vi "Get Cache Path.vi"(8 "error in (no error)":errorcluster, 11 "IPath Getter in":refnum<class "IPath Getter.lvclass">) -> (0 "error out":errorcluster, 2 "Path":path)   [LabVIEW 2020, in "IPath Getter.lvclass"]
doc: "Definition of input/output parameters for <b>Get Cache Path</b> implementation."
uses:
  IPath Getter.lvclass
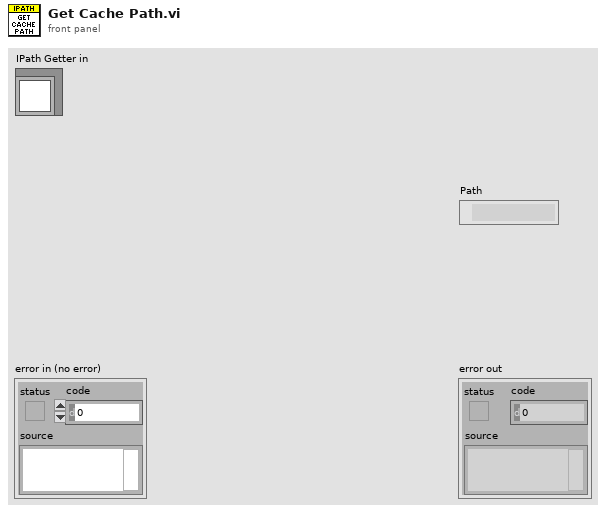
[diagram p1: front panel]
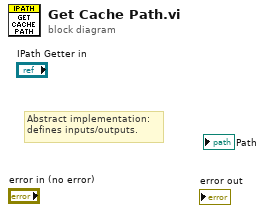
[diagram p0: block diagram]
diagram:
  # "Abstract implementation:\ndefines inputs/outputs."
